vi "CalculatePercentCompleted.vi"(10 "Dose (dpa)":dbl, 11 "Target Dose (dpa)":dbl) -> (2 "Complete?":bool, 3 "Percent Complete (%)":dbl)   [LabVIEW 2012]
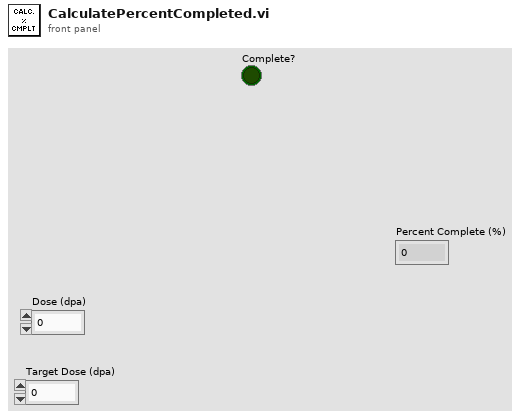
[diagram p1: front panel]
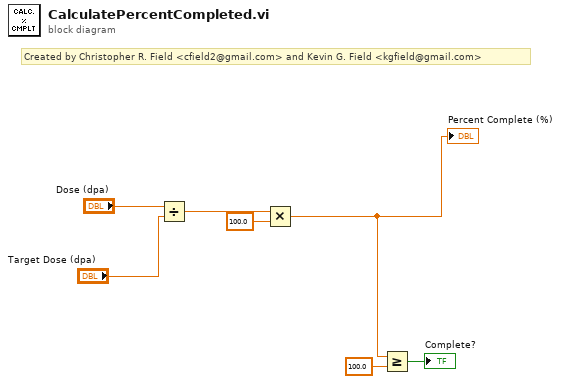
[diagram p0: block diagram]
diagram:
  # "Created by Christopher R. Field <cfield2@gmail.com> and Kevin G. Field <kgfield@gmail.com>"
  n1 = Divide(x="Dose (dpa)", y="Target Dose (dpa)") -> (x/y=w5:dbl)
  n2 = Multiply(x=w5, y=100.0) -> (x*y=w2:dbl)
  "Percent Complete (%)" <- w2
  n3 = Greater Or Equal?(x=w2, y=100.0) -> (x >= y?=→"Complete?":bool)
